vi "Decode DM.vi"(10 "GTIN":string, 11 "DataMatrix Text":string) -> (3 "DM CONTENT OUT":T1)   [LabVIEW 2024]
panel:
  out "DM Data":string[](array[string])
  out "DM Order":string[](array[string])
  out "Sep":string
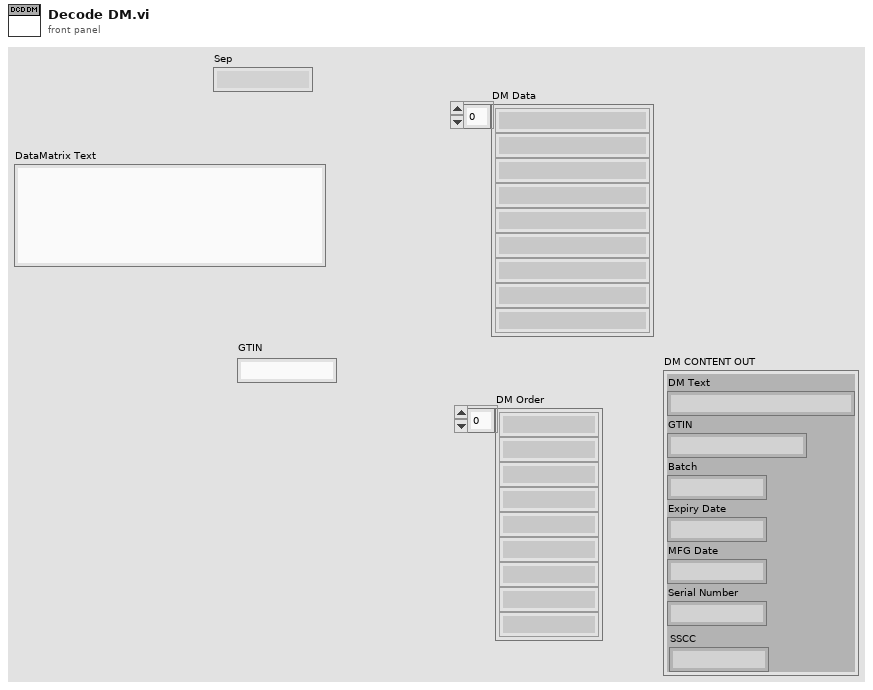
[diagram p1: front panel]
types:
  T1 = cluster{"DM Text":string, "GTIN":string, "Batch":string, "Expiry Date":string, "MFG Date":string, "Serial Number":string, "SSCC":string}
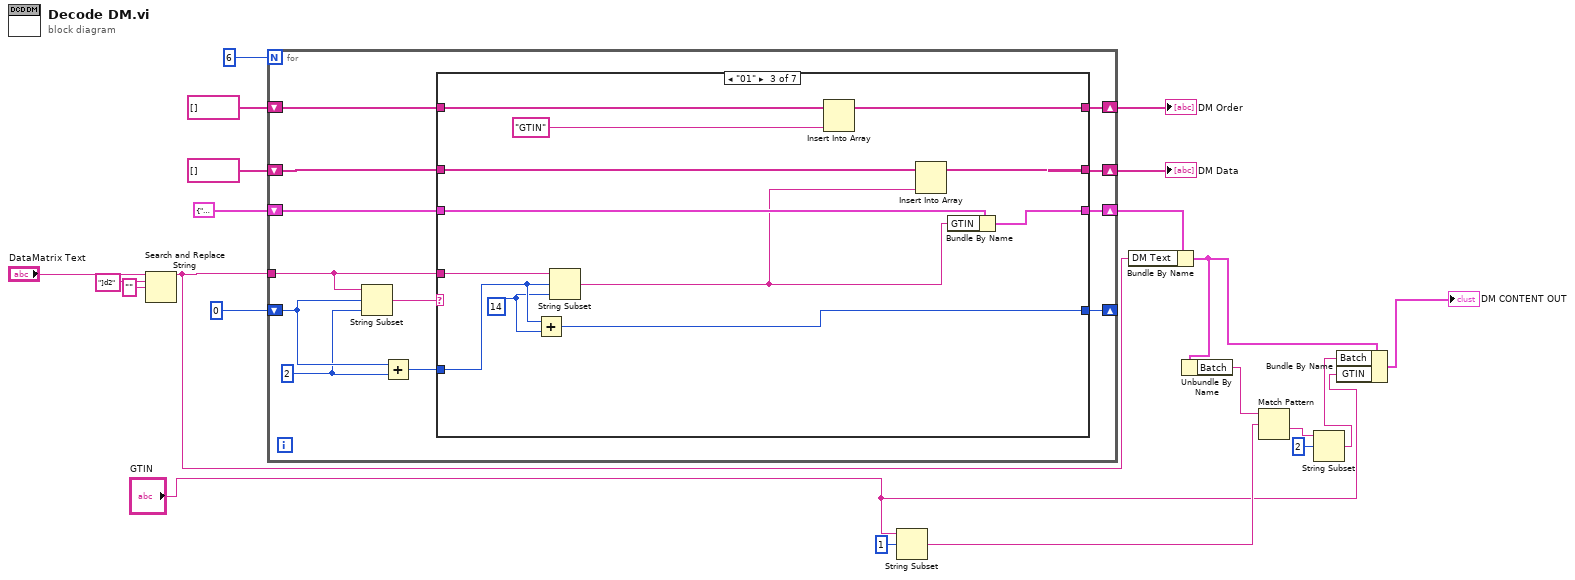
[diagram p0: block diagram]
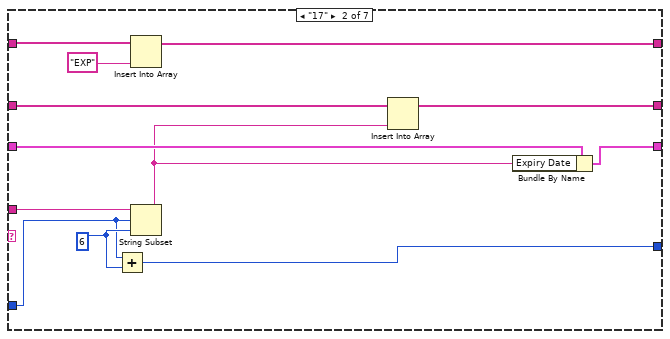
[diagram p3: hidden frame]
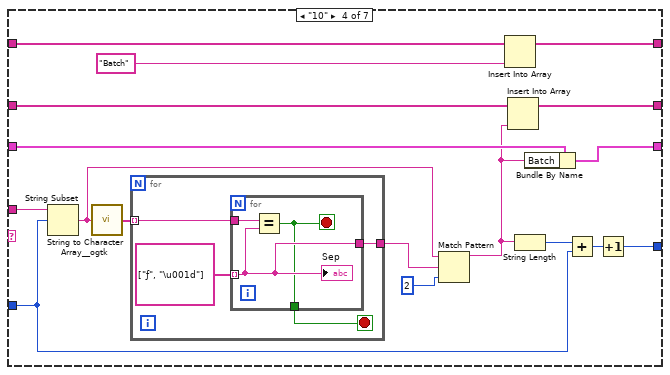
[diagram p4: hidden frame]
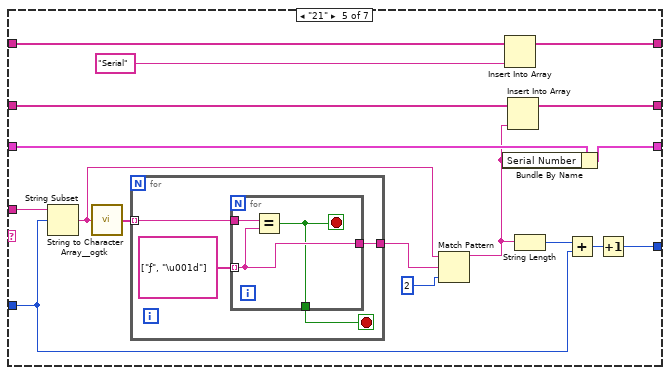
[diagram p5: hidden frame]
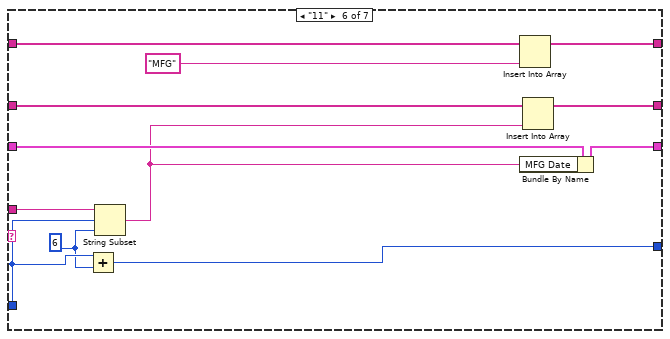
[diagram p6: hidden frame]
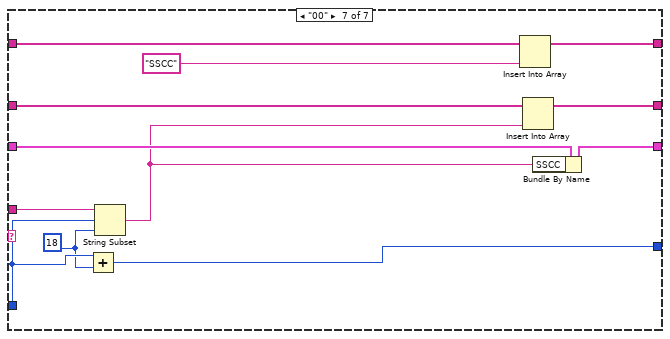
[diagram p7: hidden frame]
diagram:
  n1 = Search and Replace String(input string="DataMatrix Text", search string="]d2" ("input string"), replace string="" ("replace string (\"\")")) -> (result string=w7:string)  [unwired: 5 in, 3 out]
  n2 = for {
    N: 6 -> [_]
    tunnel: w7 -> [w31]
    shift-right: [w32] -> _
    shift-left: 0 -> [w30]
    shift-right: [w27] -> w18
    shift-left: string[] [] -> [w26]
    shift-right: [w25] -> w16
    shift-left: string[] [] -> [w24]
    shift-right: [w23] -> w15
    shift-left: T1 {"DM Text"="", "GTIN"="", "Batch"="", "Expiry Date"="", "MFG Date"="", "Serial Number"="", "SSCC"=""} ("DM CONTENT OUT") -> [w22]
    w29 = 2 ("length (rest)")
    n3 = String Subset(string=w31, offset (0)=w30, length (rest)=w29) -> (substring=w33:string)
    n4 = Add(x=w30, y=w29) -> (x+y=w28:i32)
    n5 = case shown="\"01\"" w33 {
      tunnel: w31 -> [_ w49 w61 w75 w99 w121 w133]
      tunnel: w28 -> [w35 w46 w60 w74 w98 w120 w132]
      tunnel: [w35 w47 w58 w76 w100 w118 w130] -> w32
      tunnel: [w37 w43 w55 w71 w95 w115 w127] -> w27
      tunnel: w26 -> [w37 w44 w56 w72 w96 w116 w128]
      tunnel: [w36 w41 w54 w70 w94 w113 w125] -> w25
      tunnel: w24 -> [w36 w42 w53 w69 w93 w114 w126]
      tunnel: [w34 w39 w51 w67 w91 w111 w123] -> w23
      tunnel: w22 -> [w34 w40 w52 w68 w92 w112 w124]
      frame Default {
      }
      frame "17" {
        w48 = 6 ("length (rest)")
        n6 = Add(x=w46, y=w48) -> (x+y=w47:i32)
        n7 = Insert Into Array(array=w44, new element="EXP" ("regular expression")) -> (w43:string[])  [unwired: 1 in]
        n8 = String Subset(string=w49, offset (0)=w46, length (rest)=w48) -> (substring=w38:string)
        n9 = Insert Into Array(array=w42, new element=w38) -> (w41:string[])  [unwired: 1 in]
        n10 = Bundle By Name(cluster=w40, "Expiry Date"=w38) -> (w39:T1)
      }
      frame "01" {
        w59 = 14 ("length (rest)")
        n11 = Add(x=w60, y=w59) -> (x+y=w58:i32)
        n12 = String Subset(string=w61, offset (0)=w60, length (rest)=w59) -> (substring=w50:string)
        n13 = Insert Into Array(array=w56, new element="GTIN" ("regular expression")) -> (w55:string[])  [unwired: 1 in]
        n14 = Insert Into Array(array=w53, new element=w50) -> (w54:string[])  [unwired: 1 in]
        n15 = Bundle By Name(cluster=w52, "GTIN"=w50) -> (w51:T1)
      }
      frame "10" {
        n16 = String Subset(string=w75, offset (0)=w74) -> (substring=w63:string)  [unwired: 1 in]
        n17 = call "String to Character Array__ogtk.vi"("Input String"=w63) -> ("Character Array"=w66:string[])
        n18 = for {
          tunnel: w66 -> [w81] mode=indexing
          tunnel: [w80] -> w64
          stop <- w79 stop-if-true
          n19 = for {
            tunnel: string[] ["ƒ", "\u001d"] -> [w84] mode=indexing
            tunnel: w81 -> [w85]
            tunnel: [w84] -> w80
            tunnel: [w83] -> w79
            stop <- w83 stop-if-true
            n20 = Equal?(x=w85, y=w84) -> (x = y?=w83:bool)
            "Sep" <- w84
          }
        }
        n21 = Match Pattern(string=w63, regular expression=w64, offset (0)=2) -> (before substring=w62:string)  [unwired: 3 out]
        n22 = Insert Into Array(array=w72, new element="Batch" ("regular expression")) -> (w71:string[])  [unwired: 1 in]
        n23 = Insert Into Array(array=w69, new element=w62) -> (w70:string[])  [unwired: 1 in]
        n24 = String Length(string=w62) -> (length=w77:i32)
        n25 = Bundle By Name(cluster=w68, "Batch"=w62) -> (w67:T1)
        n26 = Add(x=w77, y=w74) -> (x+y=w78:i32)
        n27 = Increment(x=w78) -> (x+1=w76:i32)
      }
      frame "21" {
        n28 = String Subset(string=w99, offset (0)=w98) -> (substring=w87:string)  [unwired: 1 in]
        n29 = call "String to Character Array__ogtk.vi"("Input String"=w87) -> ("Character Array"=w90:string[])
        n30 = for {
          tunnel: w90 -> [w105] mode=indexing
          tunnel: [w104] -> w88
          stop <- w103 stop-if-true
          n31 = for {
            tunnel: string[] ["ƒ", "\u001d"] -> [w108] mode=indexing
            tunnel: w105 -> [w109]
            tunnel: [w108] -> w104
            tunnel: [w107] -> w103
            stop <- w107 stop-if-true
            n32 = Equal?(x=w109, y=w108) -> (x = y?=w107:bool)
          }
        }
        n33 = Match Pattern(string=w87, regular expression=w88, offset (0)=2) -> (before substring=w86:string)  [unwired: 3 out]
        n34 = Bundle By Name(cluster=w92, "Serial Number"=w86) -> (w91:T1)
        n35 = Insert Into Array(array=w96, new element="Serial" ("regular expression")) -> (w95:string[])  [unwired: 1 in]
        n36 = Insert Into Array(array=w93, new element=w86) -> (w94:string[])  [unwired: 1 in]
        n37 = String Length(string=w86) -> (length=w101:i32)
        n38 = Add(x=w101, y=w98) -> (x+y=w102:i32)
        n39 = Increment(x=w102) -> (x+1=w100:i32)
      }
      frame "11" {
        w119 = 6 ("length (rest)")
        n40 = Add(x=w120, y=w119) -> (x+y=w118:i32)
        n41 = String Subset(string=w121, offset (0)=w120, length (rest)=w119) -> (substring=w110:string)
        n42 = Insert Into Array(array=w116, new element="MFG" ("regular expression")) -> (w115:string[])  [unwired: 1 in]
        n43 = Bundle By Name(cluster=w112, "MFG Date"=w110) -> (w111:T1)
        n44 = Insert Into Array(array=w114, new element=w110) -> (w113:string[])  [unwired: 1 in]
      }
      frame "00" {
        w131 = 18 ("length (rest)")
        n45 = Add(x=w132, y=w131) -> (x+y=w130:i32)
        n46 = String Subset(string=w133, offset (0)=w132, length (rest)=w131) -> (substring=w122:string)
        n47 = Insert Into Array(array=w128, new element="SSCC" ("regular expression")) -> (w127:string[])  [unwired: 1 in]
        n48 = Insert Into Array(array=w126, new element=w122) -> (w125:string[])  [unwired: 1 in]
        n49 = Bundle By Name(cluster=w124, "SSCC"=w122) -> (w123:T1)
      }
    }
  }
  "DM Order" <- w18
  "DM Data" <- w16
  n50 = String Subset(string="GTIN", offset (0)=1) -> (substring=w2:string)  [unwired: 1 in]
  n51 = Bundle By Name(cluster=w15, "DM Text"=w7) -> (w9:T1)
  n52 = Unbundle By Name(w9) -> ("Batch"=w10:string)
  n53 = Match Pattern(string=w10, regular expression=w2) -> (after substring=w6:string)  [unwired: 1 in, 3 out]
  n54 = String Subset(string=w6, offset (0)=2) -> (substring=w4:string)  [unwired: 1 in]
  n55 = Bundle By Name(cluster=w9, "Batch"=w4, "GTIN"="GTIN") -> (→"DM CONTENT OUT":T1)
